vi "updateContainerElement.vi"(9 "elementName":string, 10 "elementValue":variant, 11 "Container in":variant) -> (3 "Container out":variant)   [LabVIEW 2025, in "ObserverClass.lvlib"]
uses:
  6e2cd329-805c-4cd3-8e9e-2e4c2aacc9ac.vi
  ObserverClass.lvlib
  <vilib>/PNR/LabVIEW Composition/Composition/Composition.lvlib
  <vilib>/Utility/Data Type/NI_Data Type.lvlib
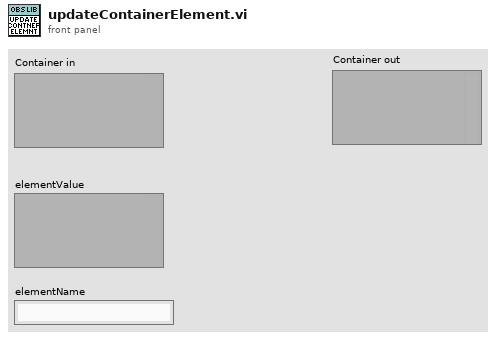
[diagram p1: front panel]
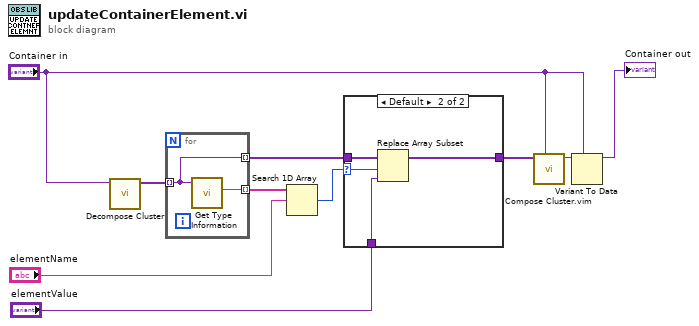
[diagram p0: block diagram]
diagram:
  n1 = call <vilib>:"Decompose Cluster.vi"("Variant Cluster"="Container in") -> ("Cluster Elements"=w9:variant[])  [unwired: 9 in, 1 out]
  n2 = for {
    tunnel: w9 -> [w11] mode=indexing
    tunnel: [w12] -> w8 mode=indexing
    tunnel: [w11] -> w6 mode=indexing
    n3 = call <vilib>:"Get Type Information.vi"("variant"=w11) -> ("name"=w12:string)  [unwired: 6 in, 4 out]
  }
  n4 = Search 1D Array(1D array=w8, element="elementName") -> (index of element=w5:i32)  [unwired: 1 in]
  n5 = case shown="Default" w5 {
    selector: w5 -> [_ w16]
    tunnel: w6 -> [w13 w17]
    tunnel: [w13 w15] -> w4
    tunnel: "elementValue" -> [_ w14]
    frame -1 {
    }
    frame Default {
      n6 = Replace Array Subset "Replace Array Subset"(array=w17, new element=w14, index=w16) -> (w15:variant[])
    }
  }
  n7 = call "Compose Cluster.vim"("Type"="Container in", "Elements"=w4) -> ("Cluster"=w10:variant)  [unwired: 8 in, 1 out]
  n8 = Variant To Data(type="Container in", Variant=w10) -> (data=→"Container out":variant)  [unwired: 1 in, 1 out]
